vi "Graph v0.1.vi"() -> ()   [LabVIEW 2017]
uses:
  <vilib>/Analysis/3filter.llb/Filter Passband Type.ctl
  <vilib>/Analysis/3filter.llb/Filter Structure Type.ctl
  <vilib>/Analysis/3filter.llb/Zero Phase Filter (DBL).vi
  <vilib>/Analysis/NI_AALBase.lvlib
  <vilib>/Analysis/NI_AAL_SigProc.lvlib
panel:
  out "Locations":dbl[](array[numeric])
  in  "peaks/valleys":enum32{"Peaks", "Valleys"}(ring)
  in  "width":i32=3 min=3
  in  "threshold":dbl format="%0.2f"
  out "Waveform Graph 7":dbl[](graph)
  in  "sampling freq: fs 2":dbl=1000.0 format="%#_13g"
  in  "low cutoff freq: fl 2":dbl=50.0 format="%#_13g"
  in  "order 2":i32=6
  in  "filter type 2":T1
  in  "filter structure option 2":T2=10 items=["IIR 2nd Order"=0, "IIR 4th Order"=1, "Auto Select"=10]
  in  "high cutoff freq: fh 2":dbl=0.45 format="%0.3f"
  out "Manual Graph 2":dbl[][](graph)
  out "Waveform Graph 6":dbl[](graph)
  in  "high cutoff freq: fh":dbl=0.45 format="%0.3f"
  in  "filter structure option":T2=10 items=["IIR 2nd Order"=0, "IIR 4th Order"=1, "Auto Select"=10]
  in  "filter type":T1
  in  "Manual Graph":dbl[][](graph)
  in  "Waveform Graph 5":dbl[][](graph)=array5x1073[5365 elements]
  in  "order":i32=6
  in  "low cutoff freq: fl":dbl=50.0 format="%#_13g"
  in  "sampling freq: fs":dbl=1000.0 format="%#_13g"
  in  "length":i32
  in  "index":i32
  out "XY Graph":cluster{dbl[], "Filtered X":dbl[]}[](graph)
  out "Waveform Graph 4":dbl[](graph)
  out "Waveform Graph 3":dbl[](graph)
  out "Waveform Graph 2":dbl[](graph)
  in  "Waveform Graph":dbl[][](graph)=array5x68100[340500 elements]
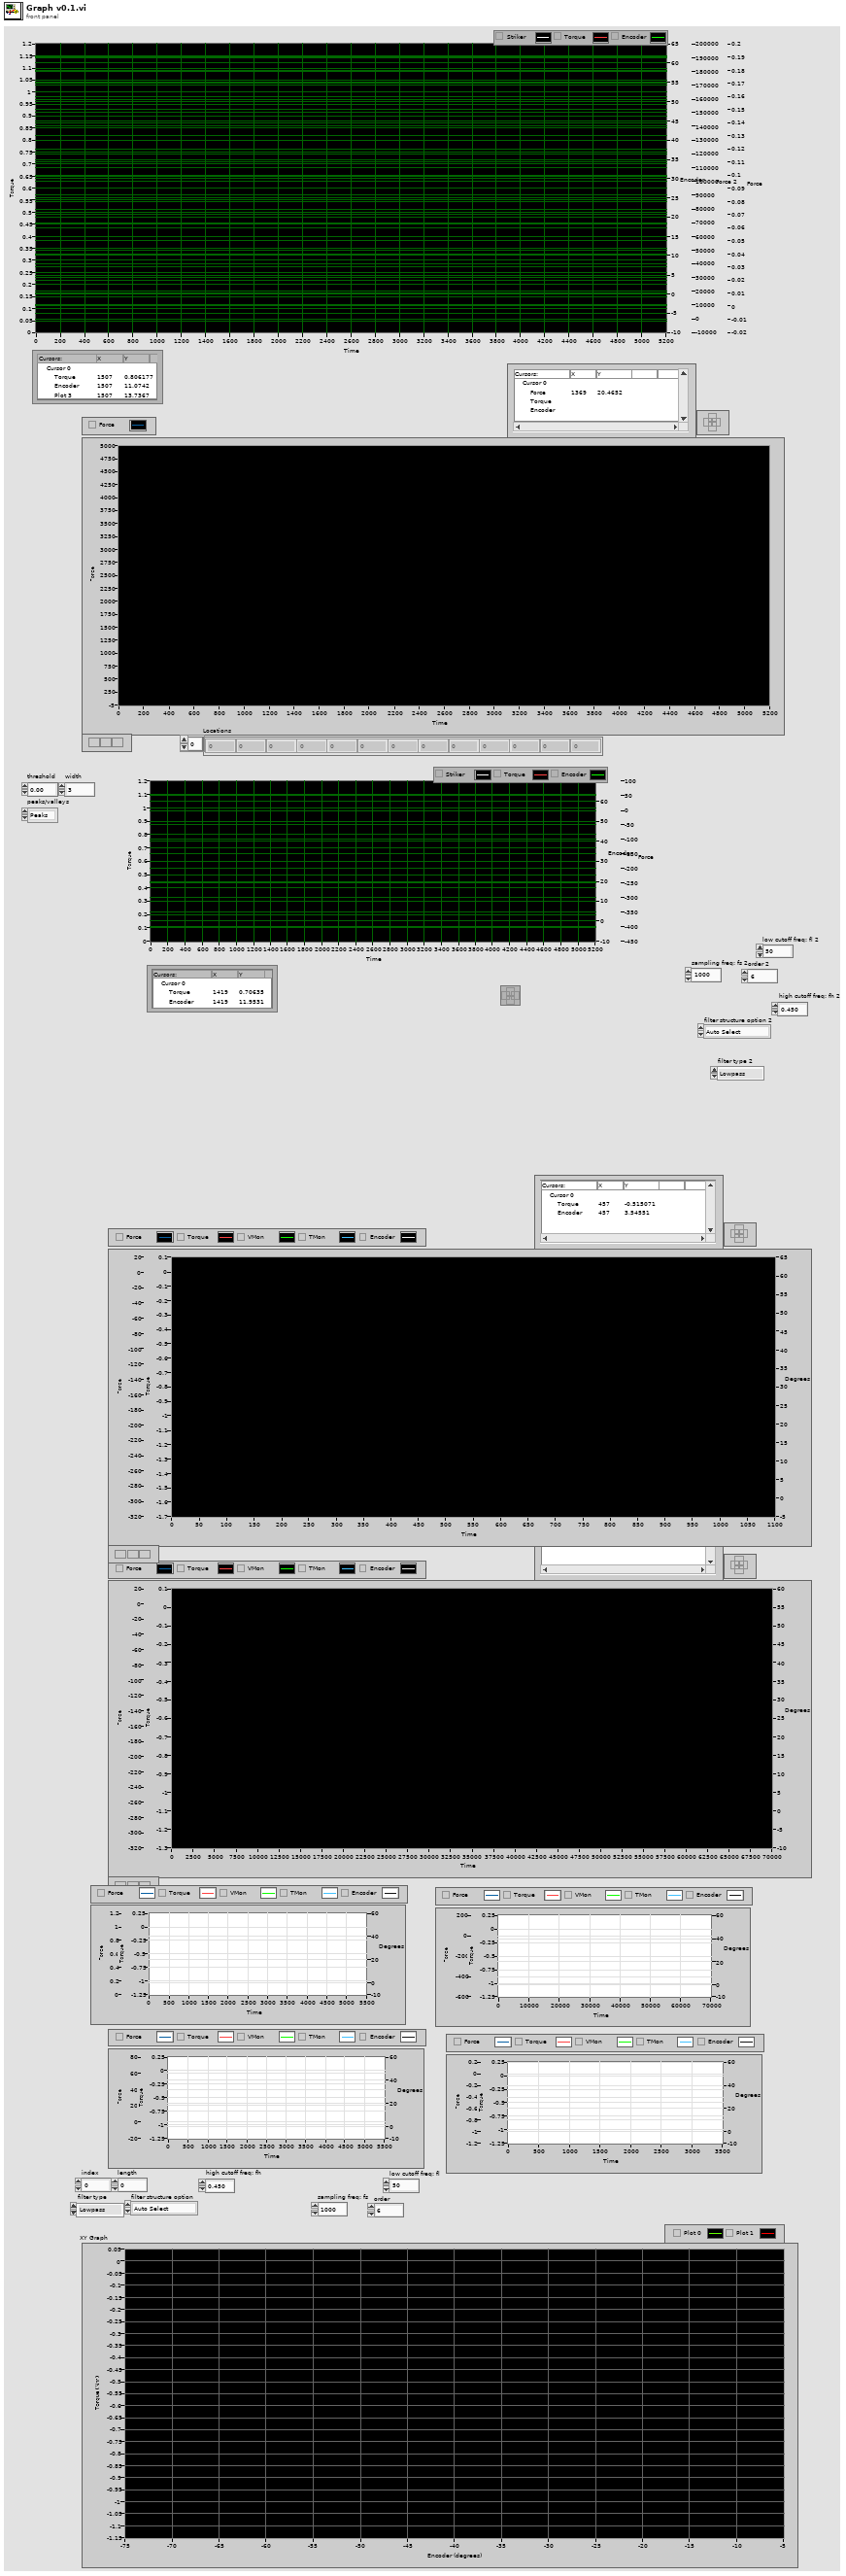
[diagram p1: front panel]
types:
  T1 = typedef "NI_AALBase.lvlib/Filter Passband Type.ctl" = enum32{"Lowpass", "Highpass", "Bandpass", "Bandstop"}
  T2 = typedef "NI_AALBase.lvlib/Filter Structure Type.ctl" = u16
  T3 = cluster{"filter structure":enum32{"IIR 2nd Order", "IIR 4th Order"}, "Reverse Coefficients":dbl[], "Forward Coefficients":dbl[]}
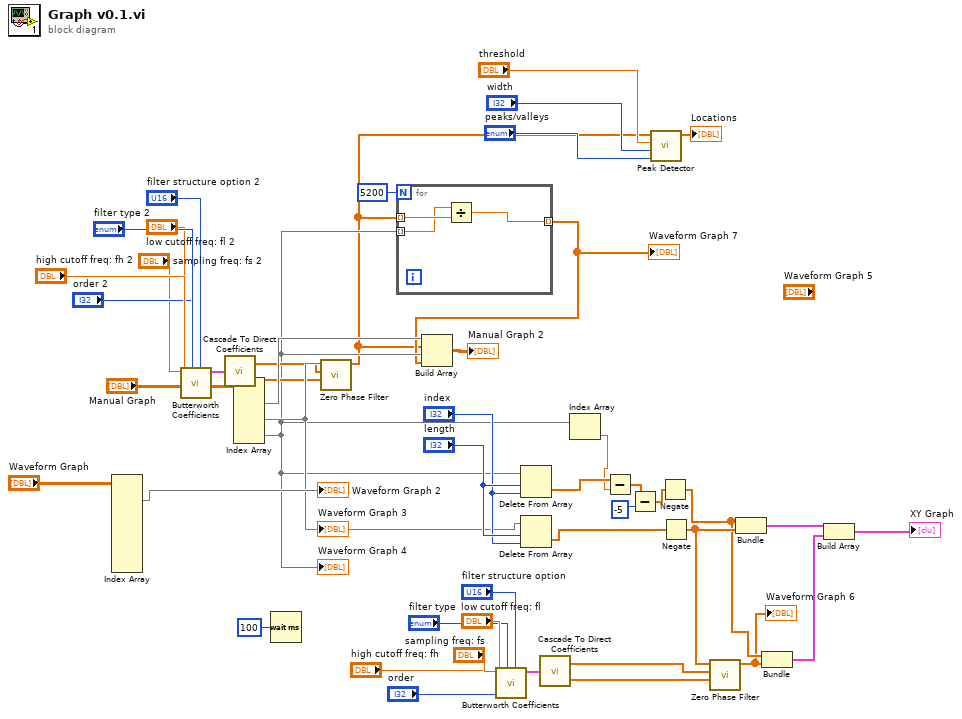
[diagram p0: block diagram]
diagram:
  n1 = Index Array(array="Waveform Graph") -> (element #1=→"Waveform Graph 2":dbl[])  [unwired: 10 in, 4 out]
  n2 = call <vilib>:"Butterworth Coefficients.vi"("filter structure option"="filter structure option 2", "order"="order 2", "filter type"="filter type 2", "low cutoff freq: fl"="low cutoff freq: fl 2", "high cutoff freq: fh"="high cutoff freq: fh 2", "sampling freq: fs"="sampling freq: fs 2") -> ("IIR Filter Cluster"=w15:T3)  [unwired: 4 in, 1 out]
  n3 = call <vilib>:"Cascade To Direct Coefficients.vi"("IIR Filter Cluster"=w15) -> ("Reverse Coefficients"=w11:dbl[], "Forward Coefficients"=w10:dbl[])
  n4 = Index Array(array="Manual Graph") -> (element #1=w20:dbl[], element #2=w19:dbl[], element #3=w8:dbl[])  [unwired: 6 in]
  "Waveform Graph 3" <- w19
  "Waveform Graph 4" <- w8
  n5 = Wait (ms)(milliseconds to wait=u32 100) -> ()  [unwired: 1 out]
  n6 = call-poly <vilib>:"Zero Phase Filter.vi"("Forward Coefficients"=w10, "Reverse Coefficients"=w11, "X"=w19) -> ("Filtered X"=w1:dbl[])  [unwired: 7 in, 1 out]
  n7 = for {
    N: 5200 -> [_]
    tunnel: w1 -> [w50] mode=indexing
    tunnel: w8 -> [w49] mode=indexing
    tunnel: [w48] -> w6 mode=indexing
    n8 = Divide(x=w49, y=w50) -> (x/y=w48:dbl)
  }
  "Waveform Graph 7" <- w6
  n9 = Build Array(w20, w1, w8, w6) -> (→"Manual Graph 2":dbl[][])
  n10 = call <vilib>:"Butterworth Coefficients.vi"("filter structure option"="filter structure option", "order"="order", "filter type"="filter type", "low cutoff freq: fl"="low cutoff freq: fl", "high cutoff freq: fh"="high cutoff freq: fh", "sampling freq: fs"="sampling freq: fs") -> ("IIR Filter Cluster"=w38:T3)  [unwired: 4 in, 1 out]
  n11 = Delete From Array(array=w8, length="length", index="index") -> (deleted portion=w45:dbl[])  [unwired: 1 out]
  n12 = Delete From Array(array=w19, length="length", index="index") -> (deleted portion=w44:dbl[])  [unwired: 1 out]
  n13 = call <vilib>:"Cascade To Direct Coefficients.vi"("IIR Filter Cluster"=w38) -> ("Reverse Coefficients"=w37:dbl[], "Forward Coefficients"=w36:dbl[])
  n14 = Index Array(array=w8) -> (element=w29:dbl)  [unwired: 1 in]
  n15 = Subtract(x=w45, y=w29) -> (x-y=w28:dbl[])
  n16 = Subtract(x=w28, y=-5 ("Waveform")) -> (x-y=w27:dbl[])
  n17 = call <vilib>:"Peak Detector.vi"("peaks/valleys"="peaks/valleys", "width"="width", "threshold"="threshold", "X"=w1) -> ("Locations"=→"Locations":dbl[])  [unwired: 3 in, 4 out]
  n18 = Negate(x=w27) -> (-x=w34:dbl[])
  n19 = Negate(x=w44) -> (-x=w35:dbl[])
  n20 = call-poly <vilib>:"Zero Phase Filter.vi"("Forward Coefficients"=w36, "Reverse Coefficients"=w37, "X"=w35) -> ("Filtered X"=w21:dbl[])  [unwired: 7 in, 1 out]
  "Waveform Graph 6" <- w21
  n21 = Bundle(w34, w35) -> (w33:cluster{dbl[], dbl[]})  [unwired: 1 in]
  n22 = Bundle(w34, "Filtered X"=w21) -> (w32:cluster{dbl[], "Filtered X":dbl[]})  [unwired: 1 in]
  n23 = Build Array(w33, w32) -> (→"XY Graph":cluster{dbl[], "Filtered X":dbl[]}[])
